vi "Leaktest Write Config 07.vi"(4 "Config Clst":T5={"Log Dir Path"=path "\\\\spa-mu2e-network\\Files/LeakRateRawData", "File Log Sec"=30.0, "34970A Sec"=5.0, "Chart hrs1"=0.5, "Chart hrs2"=0.5, "Filnen Fmt"="%y%m%d_%H%M_MN#.txt", "Temp chans"="Dev1/Ti0, Dev1/Ti2, Dev1/Ti4", "DI Lines"="Dev1/AuxPort/Di2:3", "DO Lines"="Dev1/AuxPort/Do0:1", "VISA ID 34970A"="34970A", "Baud Rate"=enum."38400", "Time Fmt"=enum."Days"} {"Chart hrs2" format="%.1f"; "Chart hrs1" format="%.1f"; "34970A Sec" format="%.1f"; "File Log Sec" format="%.1f"}, 5 "Press Scaling":T1(array[cluster])=[{"Gain"=5.0, "Offset"=0.0, "Units"="PSI", "Channel"="101", "Name"="Fill 1"}, {"Gain"=7.5, "Offset"=-7.5, "Units"="PSI", "Channel"="102", "Name"="Ref 1"}, {"Gain"=2.0, "Offset"=0.0, "Units"="H2O", "Channel"="103", "Name"="Diff 1"}, {"Gain"=7.5, "Offset"=-7.5, "Units"="PSI", "Channel"="104", "Name"="Fill 2"}, {"Gain"=7.5, "Offset"=-7.46, "Units"="PSI", "Channel"="105", "Name"="Ref 2"}, {"Gain"=2.0, "Offset"=-0.038, "Units"="H2O", "Channel"="106", "Name"="Diff 2"}], 6 "Hdr Strings":string[](array[string])=["D/T", "Dir Path", "Log Sec", "34970 sec ", "Chart hrs1", "Chart hrs2", "Filnen Frmt", "Temp chs", "DI Lines", "DO Lines", "VISA 34970", "Baud Rate", "Time Fmt", "Setpt dC", "Gain", "Integ", "Deriv", "101 Gain", "101 Ofst", "101EU", "102 Gain", "102 Ofst", "102 EU", "103 Gain", "103Ofst", "103 EU", "104 Gain", "104 Ofst", "104 EU", "105 Gain", "105 Ofst", "105 EU", "106 Gain", "106 Ofst", "106 EU"], 7 "Control Params":T2={"Setpt C"=24.0, "PID"={" gain (Kc)"=25.0, "integral min"=5.0, "derivative min"=0.0}} {"Setpt C" format="%.2f"; "PID"."derivative min" format="%.3f"; "PID"."integral min" format="%.3f"; "PID"."gain (Kc)" format="%.3f"}, 8 "error in (no error)":errorcluster, 10 "Cfg Filename":string="Leaktest.ini", 11 "Cfg File Location":T4={"Cfg directory type"=3, "Rel Log Path"="LeakTest"} {"Cfg directory type" items=["User Home"=0, "User Desktop"=1, "User Documents"=2, "User Application Data"=3, "User Preferences"=4, "User Temporary"=5, "Public Documents"=6, "Public Application Data"=7, "Public Preferences"=8, "Public Cache"=13, "System Core Libraries"=9, "System Installed Libraries"=10, "Application Files"=11, "Boot Volume Root"=12]}) -> (0 "error out":errorcluster, 3 "Actual file path":path)   [LabVIEW 2020]
uses:
  Cfg Cluster Typedef.ctl
  System Directory Type.ctl
panel:
  out "Data Strings":string[](array[string])
  # "Don't change name or channel"
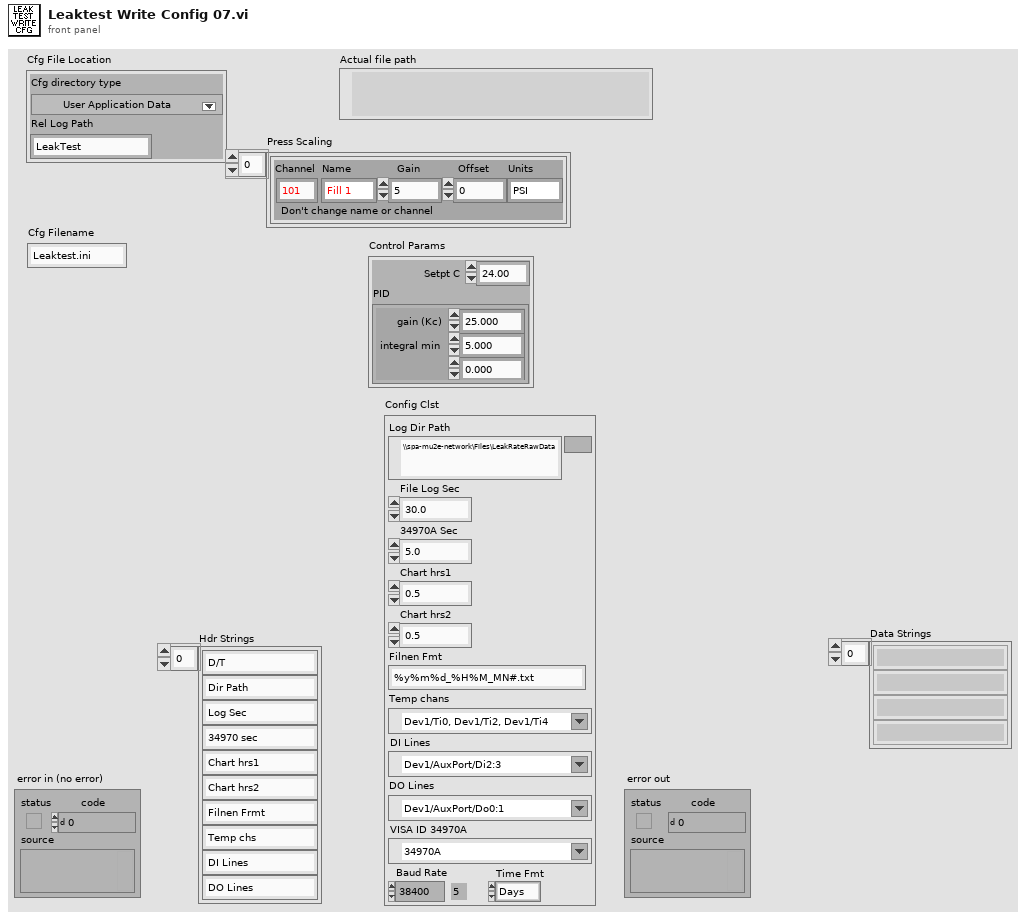
[diagram p1: front panel]
types:
  T1 = cluster{"Gain":dbl, "Offset":dbl, "Units":string, "Channel":string, "Name":string}[]
  T2 = cluster{"Setpt C":dbl, "PID":cluster{" gain (Kc)":dbl, "integral min":dbl, "derivative min":dbl}}
  T3 = typedef "System Directory Type.ctl" = i32
  T4 = cluster{"Cfg directory type":T3, "Rel Log Path":string}
  T5 = typedef "Cfg Cluster Typedef.ctl" = cluster{"Log Dir Path":path, "File Log Sec":dbl, "34970A Sec":dbl, "Chart hrs1":dbl, "Chart hrs2":dbl, "Filnen Fmt":string, "Temp chans":refnum<k21>, "DI Lines":refnum<k21>, "DO Lines":refnum<k21>, "VISA ID 34970A":refnum<visa-resource-name>, "Baud Rate":enum16{"1200", "2400", "4800", "9600", "19200", "38400", "57600", "115200"}, "Time Fmt":enum16{"H:M:S", "Days", "Secs"}}
  T6 = enum16{"1200", "2400", "4800", "9600", "19200", "38400", "57600", "115200"}
  T7 = cluster{"Press Scaling[0]":cluster{"Gain":dbl, "Offset":dbl, "Units":string, "Channel":string, "Name":string}, "Press Scaling[1]":cluster{"Gain":dbl, "Offset":dbl, "Units":string, "Channel":string, "Name":string}, "Press Scaling[2]":cluster{"Gain":dbl, "Offset":dbl, "Units":string, "Channel":string, "Name":string}, "Press Scaling[3]":cluster{"Gain":dbl, "Offset":dbl, "Units":string, "Channel":string, "Name":string}, "Press Scaling[4]":cluster{"Gain":dbl, "Offset":dbl, "Units":string, "Channel":string, "Name":string}, "Press Scaling[5]":cluster{"Gain":dbl, "Offset":dbl, "Units":string, "Channel":string, "Name":string}, "Press Scaling[6]":cluster{"Gain":dbl, "Offset":dbl, "Units":string, "Channel":string, "Name":string}, "Press Scaling[7]":cluster{"Gain":dbl, "Offset":dbl, "Units":string, "Channel":string, "Name":string}, "Press Scaling[8]":cluster{"Gain":dbl, "Offset":dbl, "Units":string, "Channel":string, "Name":string}}
  T8 = cluster{" gain (Kc)":dbl, "integral min":dbl, "derivative min":dbl}
  T9 = cluster{"Gain":dbl, "Offset":dbl, "Units":string, "Channel":string, "Name":string}
  T10 = cluster{" gain (Kc)":string, "integral min":string, "derivative min":string}
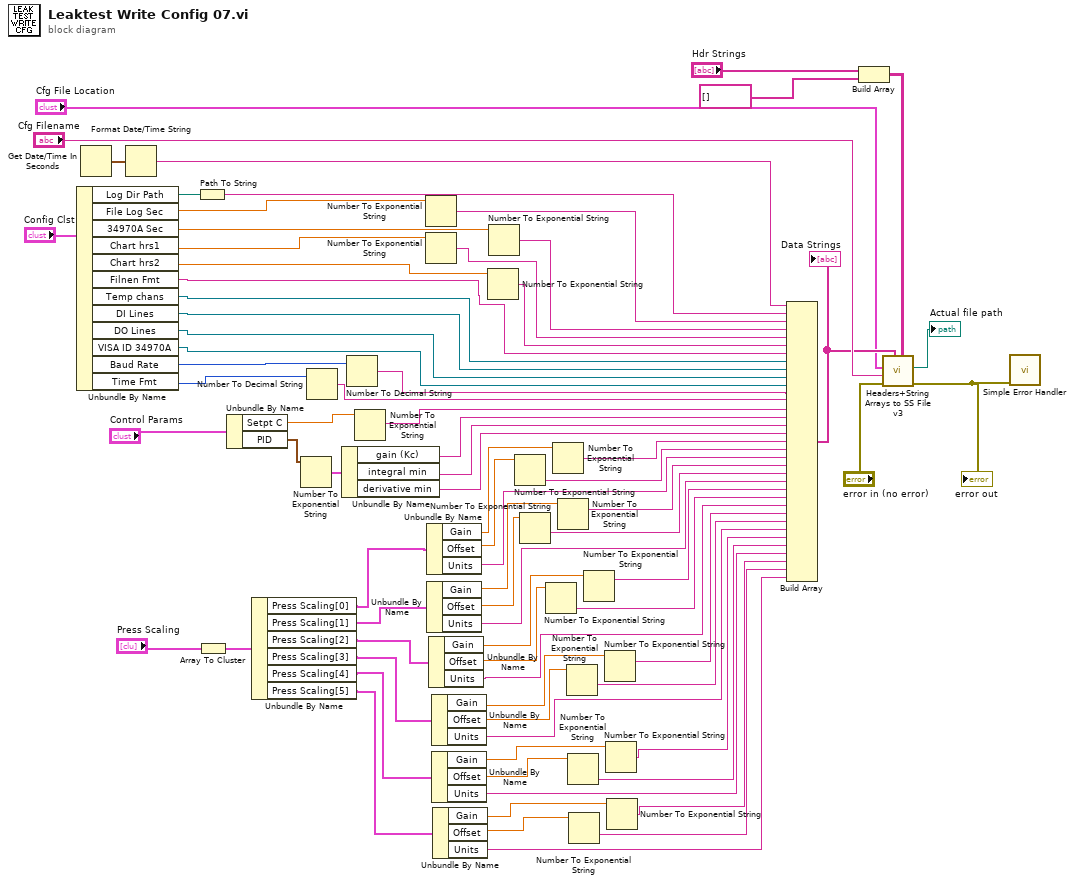
[diagram p0: block diagram]
diagram:
  n1 = Unbundle By Name("Config Clst") -> ("Log Dir Path"=w4:path, "File Log Sec"=w75:dbl, "34970A Sec"=w74:dbl, "Chart hrs1"=w73:dbl, "Chart hrs2"=w72:dbl, "Filnen Fmt"=w13:string, "Temp chans"=w12:refnum<k21>, "DI Lines"=w11:refnum<k21>, "DO Lines"=w10:refnum<k21>, "VISA ID 34970A"=w9:refnum<visa-resource-name>, "Baud Rate"=w65:T6, "Time Fmt"=w7:enum16{"H:M:S", "Days", "Secs"})
  n2 = Get Date/Time In Seconds() -> (seconds since 1Jan1904=w77:timestamp)
  n3 = Format Date/Time String(seconds (now)=w77) -> (date/time string=w2:string)  [unwired: 2 in]
  n4 = Path To String(path=w4) -> (string=w1:string)
  n5 = Array To Cluster(array="Press Scaling") -> (cluster=w66:T7)
  n6 = Unbundle By Name("Control Params") -> ("Setpt C"=w64:dbl, "PID"=w62:T8)
  n7 = Unbundle By Name(w66) -> ("Press Scaling[0]"=w34:T9, "Press Scaling[1]"=w33:T9, "Press Scaling[2]"=w32:T9, "Press Scaling[3]"=w31:T9, "Press Scaling[4]"=w30:T9, "Press Scaling[5]"=w29:T9)
  n8 = Number To Exponential String(number=w62) -> (E-format string=w61:T10)  [unwired: 3 in]
  n9 = Number To Decimal String(number=w7) -> (decimal integer string=w6:string)  [unwired: 1 in]
  n10 = Unbundle By Name(w61) -> ("gain (Kc)"=w60:string, "integral min"=w59:string, "derivative min"=w58:string)
  n11 = Number To Decimal String(number=w65) -> (decimal integer string=w8:string)  [unwired: 1 in]
  n12 = Number To Exponential String(number=w64) -> (E-format string=w63:string)  [unwired: 3 in]
  n13 = Number To Exponential String(number=w75) -> (E-format string=w17:string)  [unwired: 3 in]
  n14 = Number To Exponential String(number=w73) -> (E-format string=w15:string)  [unwired: 3 in]
  n15 = Unbundle By Name(w34) -> ("Gain"=w57:dbl, "Offset"=w56:dbl, "Units"=w53:string)
  n16 = Unbundle By Name(w33) -> ("Gain"=w52:dbl, "Offset"=w51:dbl, "Units"=w48:string)
  n17 = Unbundle By Name(w32) -> ("Gain"=w47:dbl, "Offset"=w46:dbl, "Units"=w43:string)
  n18 = Unbundle By Name(w31) -> ("Gain"=w42:dbl, "Offset"=w41:dbl, "Units"=w26:string)
  n19 = Unbundle By Name(w30) -> ("Gain"=w40:dbl, "Offset"=w39:dbl, "Units"=w23:string)
  n20 = Unbundle By Name(w29) -> ("Gain"=w38:dbl, "Offset"=w37:dbl, "Units"=w20:string)
  n21 = Number To Exponential String(number=w72) -> (E-format string=w14:string)  [unwired: 3 in]
  n22 = Number To Exponential String(number=w74) -> (E-format string=w16:string)  [unwired: 3 in]
  n23 = Number To Exponential String(number=w56) -> (E-format string=w54:string)  [unwired: 3 in]
  n24 = Number To Exponential String(number=w51) -> (E-format string=w49:string)  [unwired: 3 in]
  n25 = Number To Exponential String(number=w46) -> (E-format string=w44:string)  [unwired: 3 in]
  n26 = Number To Exponential String(number=w57) -> (E-format string=w55:string)  [unwired: 3 in]
  n27 = Number To Exponential String(number=w52) -> (E-format string=w50:string)  [unwired: 3 in]
  n28 = Number To Exponential String(number=w41) -> (E-format string=w27:string)  [unwired: 3 in]
  n29 = Number To Exponential String(number=w39) -> (E-format string=w24:string)  [unwired: 3 in]
  n30 = Number To Exponential String(number=w37) -> (E-format string=w21:string)  [unwired: 3 in]
  n31 = Number To Exponential String(number=w47) -> (E-format string=w45:string)  [unwired: 3 in]
  n32 = Number To Exponential String(number=w42) -> (E-format string=w28:string)  [unwired: 3 in]
  n33 = Number To Exponential String(number=w40) -> (E-format string=w25:string)  [unwired: 3 in]
  n34 = Number To Exponential String(number=w38) -> (E-format string=w22:string)  [unwired: 3 in]
  n35 = Build Array(w2, w1, w17, w16, w15, w14, w13, w12, w11, w10, w9, w8, w6, w63, w60, w59, w58, w55, w54, w53, w50, w49, w48, w45, w44, w43, w28, w27, w26, w25, w24, w23, w22, w21, w20) -> (w67:string[])
  "Data Strings" <- w67
  n36 = Build Array("Hdr Strings", string[] [] ("element")) -> (w68:string[][])
  n37 = call "Headers+String Arrays to SS File v3.vi"("Header"=w68, "1d Data String Array"=w67, "error in"="error in (no error)", "File Name"="Cfg Filename", "File Location"="Cfg File Location") -> ("error out"=w35:errorcluster, "Actual file path"=→"Actual file path":path)  [unwired: 5 in]
  "error out" <- w35
  n38 = call "Simple Error Handler.vi"("error in (no error)"=w35) -> ()  [unwired: 4 in, 5 out]
